vi "Periodic Tasks.vi"(8 "error in":errorcluster) -> ()   [LabVIEW 2013]
doc: "This VI runs in parallel to other tasks. It can contain as many user-defined periodic loops as you need. These can carry out PID or other sorts of timed response."
uses:
  <vilib>/Rock Robotics/SystemInterfaces/Utilities/FPGA_UtilitiesLED Source.ctl
  <vilib>/Rock Robotics/SystemInterfaces/Utilities/FPGA_UtilitiesLED State.ctl
  <vilib>/Rock Robotics/WPI/Joystick/WPI_JoystickGetSetRefNum.vi
  Robot Global Data.vi
  <vilib>/Rock Robotics/WPI/Relay/WPI_RelayValue.ctl
panel:
  out "JS Buttons 2":T1
  out "JS Buttons 1":T1
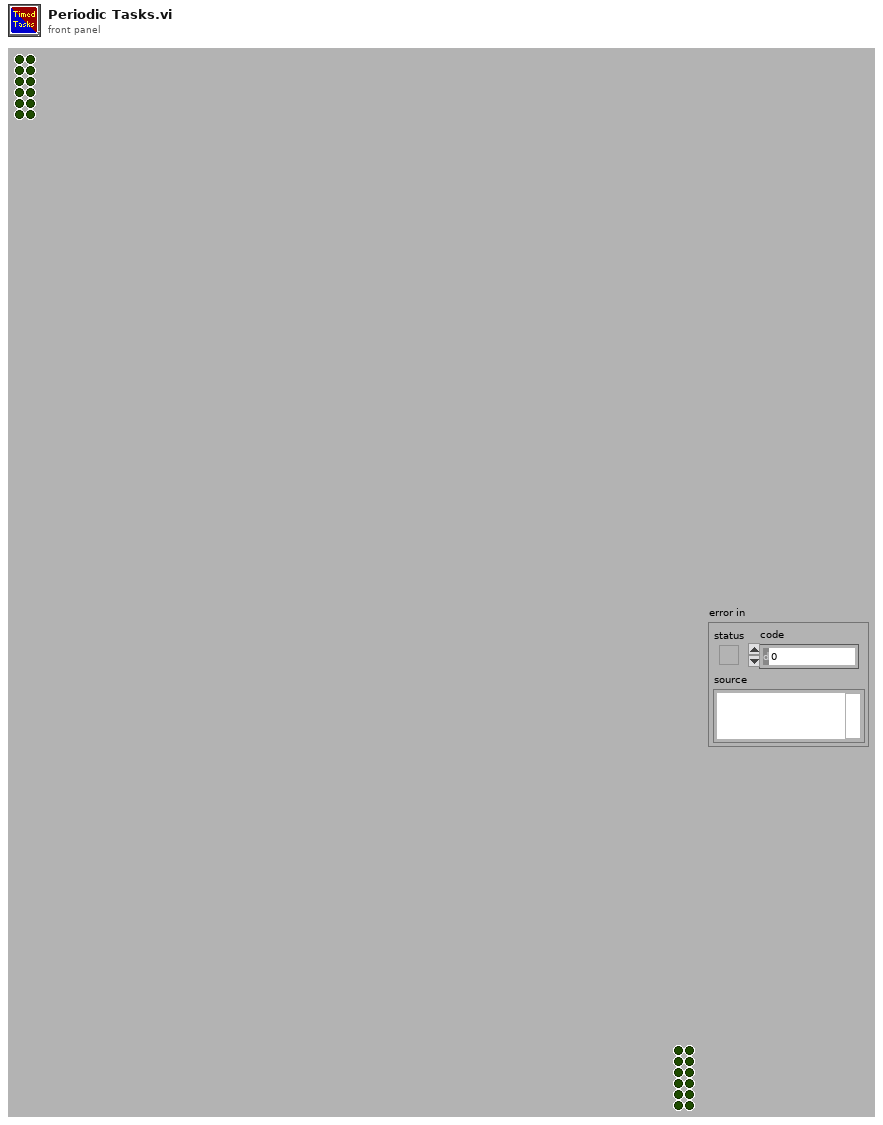
[diagram p1: front panel]
types:
  T1 = cluster{bool, bool, bool, bool, bool, bool, bool, bool, bool, bool, bool, bool}
  T2 = typedef "WPI_JoystickDevRef.ctl" = cluster{"Device":T3}
  T3 = typedef "WPI_JoystickDeviceEnum.ctl" = enum16{"USB 1", "USB 2", "USB 3", "USB 4", "Kinect 1", "Kinect 2"}
  T4 = typedef "WPI_ServoDeviceRef.ctl" = cluster{"DeviceStatus":errorcluster, "Digital Module":T5, "PWM Channel":T6, "DeadBand":T7}
  T5 = typedef "FPGA_TypedefDigitalModule.ctl" = enum16{"Digital Module 1", "Digital Module 2"}
  T6 = typedef "FPGA_DIOPWMChannel.ctl" = enum8{"PWM 1", "PWM 2", "PWM 3", "PWM 4", "PWM 5", "PWM 6", "PWM 7", "PWM 8", "PWM 9", "PWM 10", "Invalid"}
  T7 = typedef "WPI_PWMDeadband.ctl" = cluster{"Name":string, "maxPositivePwm":i32, "minPositivePwm":i32, "centerPwm":i32, "maxNegativePwm":i32, "minNegativePwm":i32, "angularRange":u16}
  T8 = typedef "WPI_MotorControlDeviceRef.ctl" = cluster{"DeviceStatus":errorcluster, "Type":enum16{"PWM", "CAN"}, "PWM":cluster{"Digital Module":T5, "PWM Channel":T6, "DeadBand":T7}, "CAN":cluster{"Device Number":u8, "Control Mode":T9, "Semaphore":T10, "Max Vout":dbl}, "Invert":bool, "TransformRef":T11, "InvTransformRef":T11}
  T9 = typedef "WPI_CANJaguar_ControlMode.ctl" = enum8{"Percent VBus", "Current", "Speed", "Position", "Voltage"}
  T10 = typedef "Semaphore RefNum" = refnum<k1>
  T11 = typedef "WPI_PWMTransform_ConPane.ctl" = refnum<vi>
  T12 = typedef "WPI_RelayDevRef.ctl" = cluster{"DevStatus":errorcluster, "Relay Channel":T13, "Digital Module":T5, "Relay Direction":T14}
  T13 = typedef "FPGA_DIORelayChannel.ctl" = enum8{"Relay 1", "Relay 2", "Relay 3", "Relay 4", "Relay 5", "Relay 6", "Relay 7", "Relay 8", "Invalid"}
  T14 = typedef "WPI_RelayDirection.ctl" = enum16{"Both directions", "Forward only", "Reverse only"}
  T15 = typedef "FPGA_UtilitiesLED State.ctl" = enum16{"Off", "On", "Toggle"}
  T16 = typedef "FPGA_UtilitiesLED Source.ctl" = enum16{"User LED", "FPGA LED"}
  T17 = typedef "WPI_RelayValue.ctl" = enum16{"Off", "On", "Forward", "Reverse"}
  T18 = typedef "WPI_JoystickButtonState.ctl" = cluster{"Button 1":bool, "Button 2":bool, "Button 3":bool, "Button 4":bool, "Button 5":bool, "Button 6":bool, "Button 7":bool, "Button 8":bool, "Button 9":bool, "Button 10":bool, "Button 11":bool, "Button 12":bool}
  T19 = cluster{"axis 1 (x)":dbl, "axis 2 (y)":dbl, "axis 3 (throttle)":dbl, "axis 4":dbl, "axis 5":dbl, "axis 6":dbl}
  T20 = typedef "WPI_DigitalInputDevRef.ctl" = cluster{"DevStatus":errorcluster, "DIO Channel":T21, "Digital Module":T5}
  T21 = typedef "FPGA_DIOChannel.ctl" = enum8{"DIO 1", "DIO 2", "DIO 3", "DIO 4", "DIO 5", "DIO 6", "DIO 7", "DIO 8", "DIO 9", "DIO 10", "DIO 11", "DIO 12", "DIO 13", "DIO 14", "Invalid"}
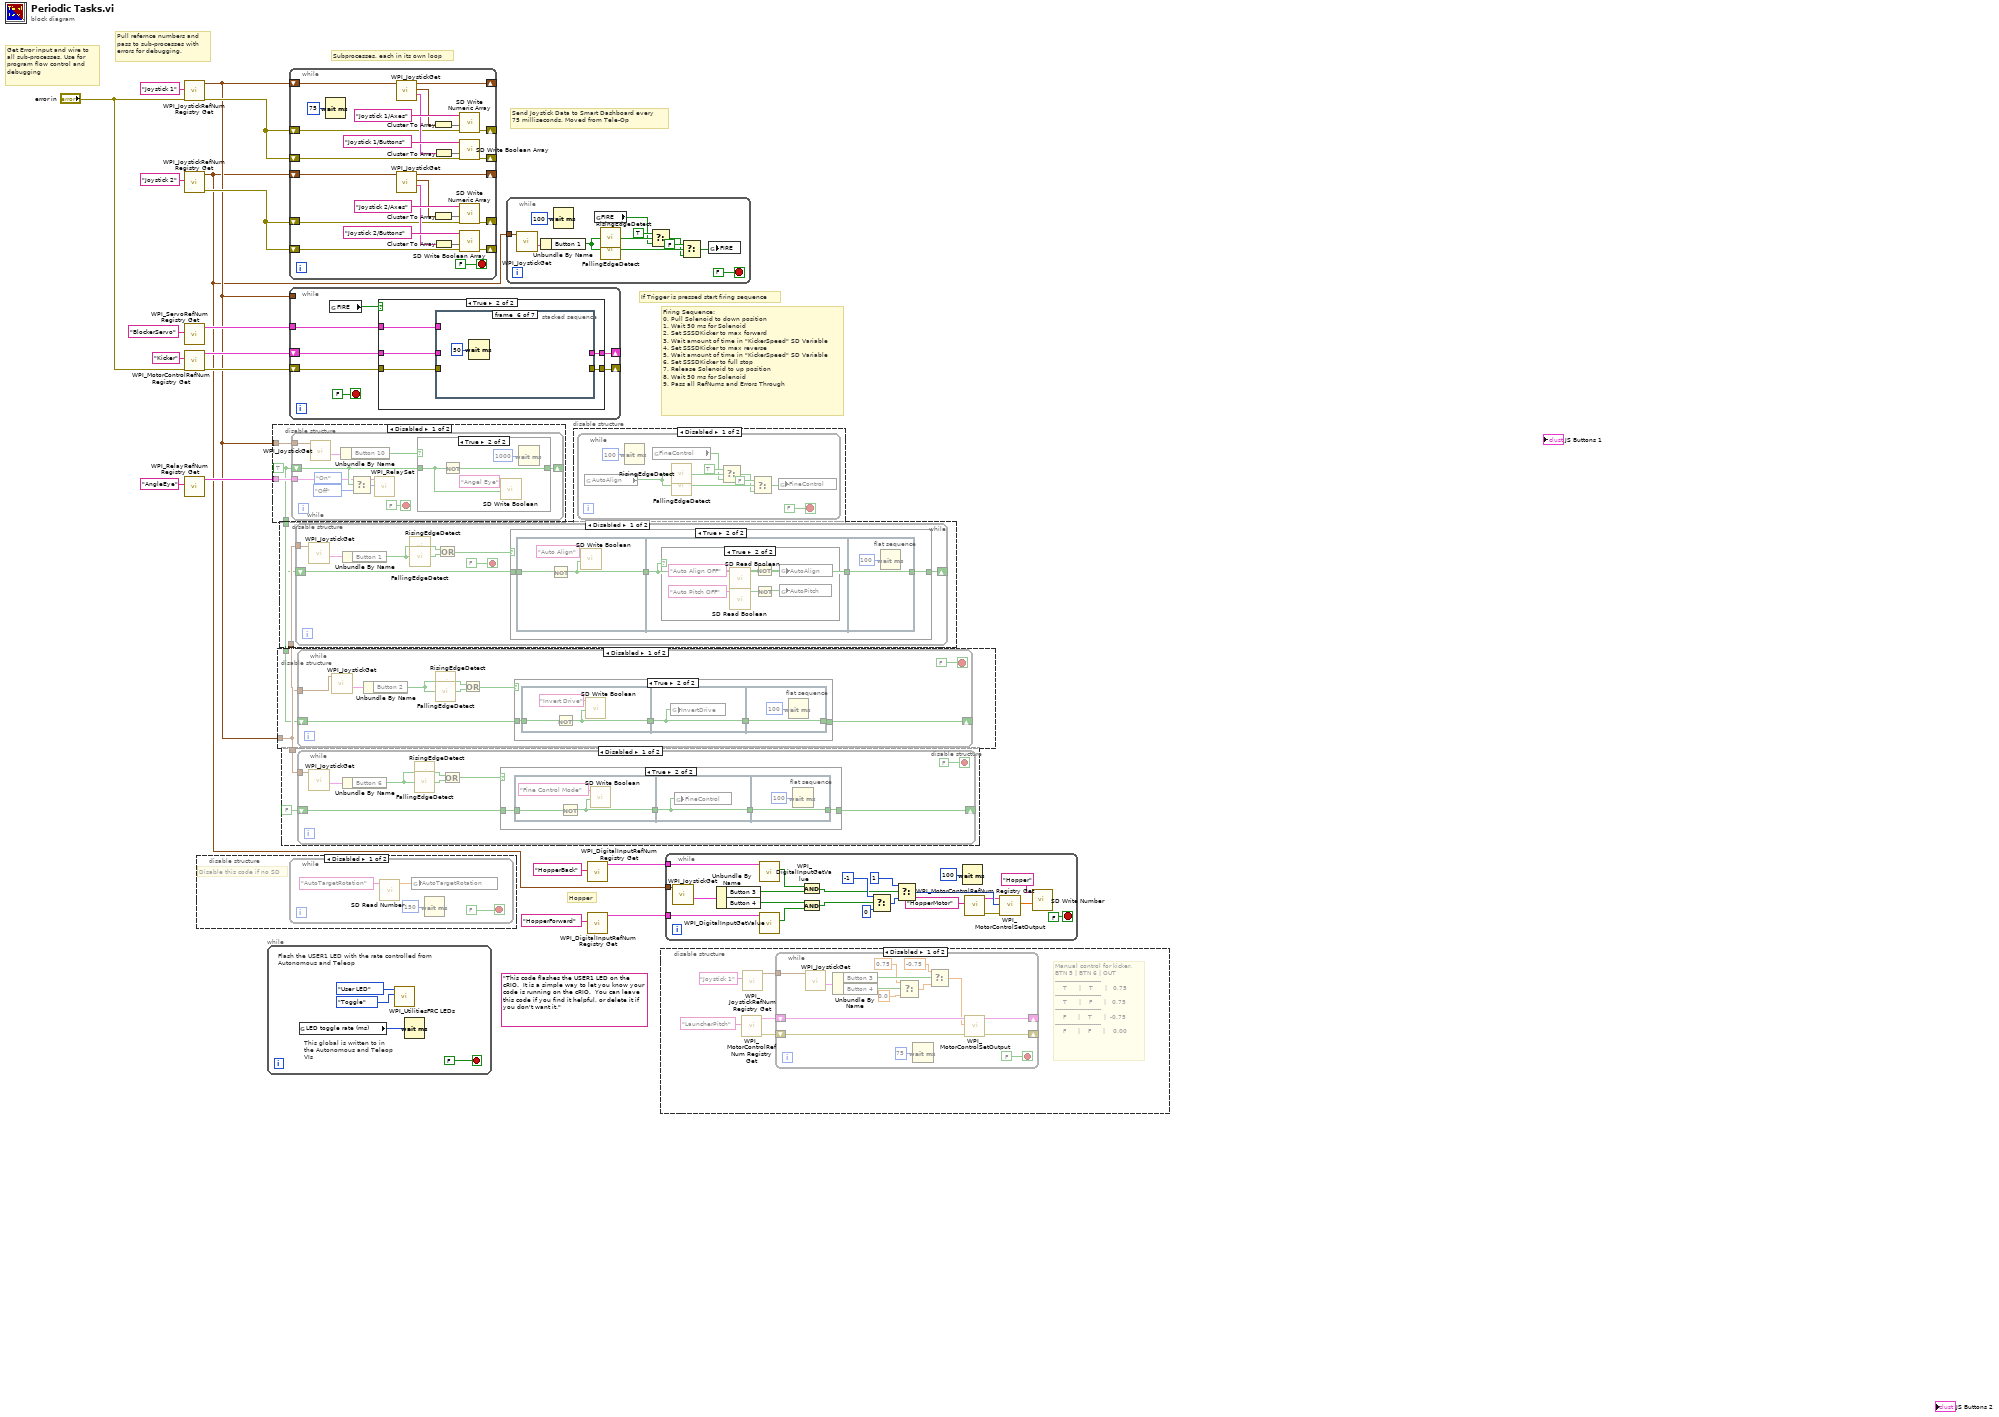
[diagram p0: block diagram]
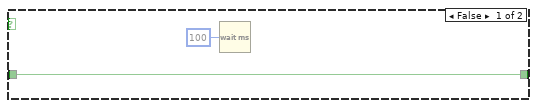
[diagram p3: hidden frame]
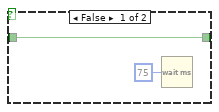
[diagram p5: hidden frame]
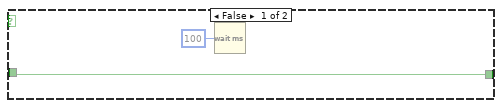
[diagram p7: hidden frame]
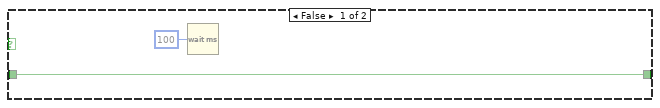
[diagram p11: hidden frame]
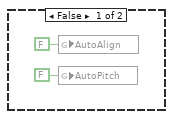
[diagram p12: hidden frame]
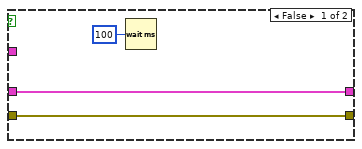
[diagram p14: hidden frame]
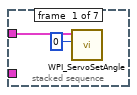
[diagram p15: hidden frame]
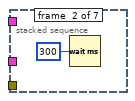
[diagram p16: hidden frame]
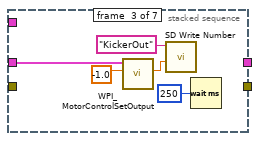
[diagram p17: hidden frame]
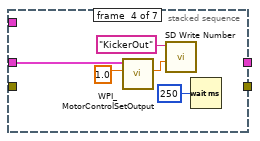
[diagram p18: hidden frame]
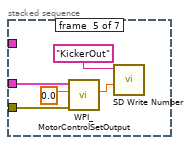
[diagram p19: hidden frame]
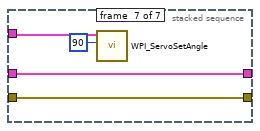
[diagram p20: hidden frame]
diagram:
  (unwired) "This code flashes the USER1 LED on the cRIO.  It is a simple way to let you know your code is running on the cRIO.  You can leave this code if you find it helpful, or delete it if you don't want it."
  # "Hopper"
  # "Firing Sequence:\n0. Pull Solenoid to down position\n1. Wait 50 ms for Solenoid\n2. Set SSSDKicker to max forward\n3. Wait amount of time in \"KickerSpeed\" SD Variable\n4. Set SSSDKicker to max reverse\n5. Wait amount of time in \"KickerSpeed\" SD Variable\n6. Set SSSDKicker to full stop\n7. Release Solenoid to up position\n8. Wait 50 ms for Solenoid\n9. Pass all RefNums and Errors Through"
  # "If Trigger is pressed start firing sequence"
  # "Subprocesses, each in its own loop"
  # "Pull refernce numbers and\npass to sub-processes with\nerrors for debugging."
  # "Get Error input and wire to\nall sub-processes. Use for\nprogram flow control and\ndebugging"
  # "Send Joystick Data to Smart Dashboard every\n75 milliseconds. Moved from Tele-Op"
  n1 = call <vilib>:"WPI_JoystickRefNum Registry Get.vi"("error in (no error)"="error in", "refnum name"="Joystick 1") -> ("error out"=w14:errorcluster, "JoystickDevRef"=w2:T2)  [unwired: 8 out]
  n2 = call <vilib>:"WPI_JoystickRefNum Registry Get.vi"("refnum name"="Joystick 2") -> ("error out"=w13:errorcluster, "JoystickDevRef"=w1:T2)  [unwired: 1 in, 8 out]
  n3 = call <vilib>:"WPI_ServoRefNum Registry Get.vi"("refnum name"="BlockerServo") -> ("ServoDeviceRef"=w9:T4)  [unwired: 9 in, 1 out]
  n4 = call <vilib>:"WPI_MotorControlRefNum Registry Get.vi"("error in (no error)"="error in", "refnum name"="Kicker") -> ("error out"=w17:errorcluster, "MotorControlDevRef"=w16:T8)  [unwired: 8 in]
  n5 = call <vilib>:"WPI_RelayRefNum Registry Get.vi"("refnum name"="AngleEye") -> ("RelayDevRef"=w11:T12)  [unwired: 9 in, 1 out]
  n6 = disable-structure shown="Disabled" {
    frame Disabled {
      # "Disable this code if no SD"
      n7 = while {
        stop <- FALSE stop-if-true
        n8 = call <vilib>:"SD Read Number.vi"("Name"="AutoTargetRotation") -> ("Numeric"=w21:dbl)  [unwired: 8 in, 2 out]
        n9 = global write "Robot Global Data.vi" "AutoTargetRotation"(w21) -> ()
        n10 = Wait (ms)(milliseconds to wait=u32 150) -> ()  [unwired: 1 out]
      }
    }
    frame Enabled {
    }
  }
  n11 = while {
    stop <- FALSE stop-if-true
    # "This global is written to in the Autonomous and Teleop VIs"
    # "Flash the USER1 LED with the rate controlled from Autonomous and Teleop"
    n12 = global read "Robot Global Data.vi" "LED toggle rate (ms)"() -> (w24:u32)
    n13 = call <vilib>:"WPI_UtilitiesFRC LEDs.vi"("State"=FPGA_UtilitiesLED_State."Toggle", "LED Type"=FPGA_UtilitiesLED_Source."User LED") -> ()  [unwired: 1 in, 9 out]
    n14 = Wait (ms)(milliseconds to wait=w24) -> ()  [unwired: 1 out]
  }
  n15 = disable-structure shown="Disabled" {
    disable-tunnel: w11 -> [w30 _]
    disable-tunnel: [w29 _] -> w3
    disable-tunnel: w2 -> [w28 _]
    frame Disabled {
      w29 = TRUE
      n16 = while {
        tunnel: w30 -> [w39]
        tunnel: w28 -> [w38]
        shift-right: [w32] -> _
        shift-left: w29 -> [w40]
        stop <- FALSE stop-if-true
        n17 = call <vilib>:"WPI_JoystickGet.vi"("JoystickDevRef"=w38) -> ("Buttons"=w33:T18)  [unwired: 4 in, 2 out]
        n18 = Unbundle By Name(w33) -> ("Button 10"=w37:bool)
        n19 = Select(t=WPI_RelayValue."On" ("RelayValue"), s=w40, f=WPI_RelayValue."Off" ("RelayValue")) -> (s? t:f=w36:T17)
        n20 = call <vilib>:"WPI_RelaySet.vi"("RelayValue"=w36, "RelayDevRef"=w39) -> ()  [unwired: 8 in, 2 out]
        n21 = case shown="True" w37 {
          tunnel: w40 -> [w41 w43]
          tunnel: [w41 w46] -> w32
          frame False {
            n22 = Wait (ms)(milliseconds to wait=u32 75) -> ()  [unwired: 1 out]
          }
          frame True {
            n23 = Not(x=w43) -> (.not. x?=w46:bool)
            n24 = call <vilib>:"SD Write Boolean.vi"("Boolean"=w43, "Name"="Angel Eye") -> ()  [unwired: 8 in, 2 out]
            n25 = Wait (ms)(milliseconds to wait=u32 1000) -> ()  [unwired: 1 out]
          }
        }
      }
    }
    frame Enabled {
    }
  }
  n26 = disable-structure shown="Disabled" {
    disable-tunnel: w3 -> [w48 _]
    disable-tunnel: w2 -> [w47 _]
    frame Disabled {
      n27 = while {
        tunnel: w47 -> [w52]
        shift-right: [w50] -> _
        shift-left: w48 -> [w49]
        stop <- FALSE stop-if-true
        n28 = call <vilib>:"WPI_JoystickGet.vi"("JoystickDevRef"=w52) -> ("Buttons"=w53:T18)  [unwired: 4 in, 2 out]
        n29 = Unbundle By Name(w53) -> ("Button 2"=w54:bool)
        n30 = call "RisingEdgeDetect.vi"("Input"=w54) -> ("Output"=w56:bool)
        n31 = call "FallingEdgeDetect.vi"("Input"=w54) -> ("Output"=w55:bool)
        n32 = Or(x=w56, y=w55) -> (x .or. y?=w57:bool)
        n33 = case shown="True" w57 {
          tunnel: [w58 w60] -> w50
          tunnel: w49 -> [w58 w61]
          frame False {
            n34 = Wait (ms)(milliseconds to wait=u32 100) -> ()  [unwired: 1 out]
          }
          frame True {
            n35 = flat-sequence {
              tunnel: w61 -> [w66]
              tunnel: [w64] -> w63
              tunnel: w63 -> [w67]
              tunnel: [w67] -> w62
              tunnel: [w69] -> w60
              tunnel: w62 -> [w69]
              frame #0 {
                n36 = Not(x=w66) -> (.not. x?=w64:bool)
                n37 = call <vilib>:"SD Write Boolean.vi"("Boolean"=w64, "Name"="Invert Drive") -> ()  [unwired: 8 in, 2 out]
              }
              frame #1 {
                n38 = global write "Robot Global Data.vi" "InvertDrive"(w67) -> ()
              }
              frame #2 {
                n39 = Wait (ms)(milliseconds to wait=u32 100) -> ()  [unwired: 1 out]
              }
            }
          }
        }
      }
    }
    frame Enabled {
    }
  }
  n40 = disable-structure shown="Disabled" {
    disable-tunnel: w2 -> [w71 _]
    disable-tunnel: w3 -> [w70 _]
    frame Disabled {
      n41 = while {
        tunnel: w71 -> [w74]
        shift-right: [w72] -> _
        shift-left: w70 -> [w80]
        stop <- FALSE stop-if-true
        n42 = call <vilib>:"WPI_JoystickGet.vi"("JoystickDevRef"=w74) -> ("Buttons"=w75:T18)  [unwired: 4 in, 2 out]
        n43 = Unbundle By Name(w75) -> ("Button 1"=w79:bool)
        n44 = call "RisingEdgeDetect.vi"("Input"=w79) -> ("Output"=w77:bool)
        n45 = call "FallingEdgeDetect.vi"("Input"=w79) -> ("Output"=w76:bool)
        n46 = Or(x=w77, y=w76) -> (x .or. y?=w78:bool)
        n47 = case shown="True" w78 {
          tunnel: w80 -> [w81 w86]
          tunnel: [w81 w85] -> w72
          frame False {
            n48 = Wait (ms)(milliseconds to wait=u32 100) -> ()  [unwired: 1 out]
          }
          frame True {
            n49 = flat-sequence {
              tunnel: w86 -> [w89]
              tunnel: [w87] -> w84
              tunnel: w84 -> [w90]
              tunnel: [w90] -> w83
              tunnel: [w100] -> w85
              tunnel: w83 -> [w100]
              frame #0 {
                n50 = Not(x=w89) -> (.not. x?=w87:bool)
                n51 = call <vilib>:"SD Write Boolean.vi"("Boolean"=w87, "Name"="Auto Align") -> ()  [unwired: 8 in, 2 out]
              }
              frame #1 {
                n52 = case shown="True" w90 {
                  frame False {
                    n53 = global write "Robot Global Data.vi" "AutoAlign"(FALSE ("AutoAlign")) -> ()
                    n54 = global write "Robot Global Data.vi" "AutoPitch"(FALSE ("AutoPitch")) -> ()
                  }
                  frame True {
                    n55 = call <vilib>:"SD Read Boolean.vi"("Name"="Auto Align OFF") -> ("Boolean"=w95:bool)  [unwired: 8 in, 2 out]
                    n56 = call <vilib>:"SD Read Boolean.vi"("Name"="Auto Pitch OFF") -> ("Boolean"=w93:bool)  [unwired: 8 in, 2 out]
                    n57 = Not(x=w95) -> (.not. x?=w96:bool)
                    n58 = Not(x=w93) -> (.not. x?=w94:bool)
                    n59 = global write "Robot Global Data.vi" "AutoAlign"(w96) -> ()
                    n60 = global write "Robot Global Data.vi" "AutoPitch"(w94) -> ()
                  }
                }
              }
              frame #2 {
                n61 = Wait (ms)(milliseconds to wait=u32 100) -> ()  [unwired: 1 out]
              }
            }
          }
        }
      }
    }
    frame Enabled {
    }
  }
  n62 = disable-structure shown="Disabled" {
    disable-tunnel: w2 -> [w101 _]
    frame Disabled {
      n63 = while {
        shift-right: [w103] -> _
        shift-left: FALSE -> [w108]
        tunnel: w101 -> [w105]
        stop <- FALSE stop-if-true
        n64 = call <vilib>:"WPI_JoystickGet.vi"("JoystickDevRef"=w105) -> ("Buttons"=w106:T18)  [unwired: 4 in, 2 out]
        n65 = Unbundle By Name(w106) -> ("Button 6"=w107:bool)
        n66 = call "RisingEdgeDetect.vi"("Input"=w107) -> ("Output"=w110:bool)
        n67 = call "FallingEdgeDetect.vi"("Input"=w107) -> ("Output"=w109:bool)
        n68 = Or(x=w110, y=w109) -> (x .or. y?=w111:bool)
        n69 = case shown="True" w111 {
          tunnel: w108 -> [w112 w114]
          tunnel: [w112 w115] -> w103
          frame False {
            n70 = Wait (ms)(milliseconds to wait=u32 100) -> ()  [unwired: 1 out]
          }
          frame True {
            n71 = flat-sequence {
              tunnel: [w119] -> w117
              tunnel: w114 -> [w118]
              tunnel: w117 -> [w121]
              tunnel: [w121] -> w116
              tunnel: [w123] -> w115
              tunnel: w116 -> [w123]
              frame #0 {
                n72 = Not(x=w118) -> (.not. x?=w119:bool)
                n73 = call <vilib>:"SD Write Boolean.vi"("Boolean"=w119, "Name"="Fine Control Mode") -> ()  [unwired: 8 in, 2 out]
              }
              frame #1 {
                n74 = global write "Robot Global Data.vi" "FineControl"(w121) -> ()
              }
              frame #2 {
                n75 = Wait (ms)(milliseconds to wait=u32 100) -> ()  [unwired: 1 out]
              }
            }
          }
        }
      }
    }
    frame Enabled {
    }
  }
  n76 = while {
    shift-right: [w140] -> _
    shift-left: w14 -> [w138]
    shift-right: [w139] -> _
    shift-left: w14 -> [w137]
    shift-right: [w136] -> _
    shift-left: w2 -> [w141]
    shift-right: [w124] -> _
    shift-left: w1 -> [w127]
    shift-right: [w126] -> _
    shift-left: w13 -> [w129]
    shift-right: [w125] -> _
    shift-left: w13 -> [w128]
    stop <- FALSE stop-if-true
    n77 = Wait (ms)(milliseconds to wait=u32 75) -> ()  [unwired: 1 out]
    n78 = call <vilib>:"WPI_JoystickGet.vi"("JoystickDevRef"=w141) -> ("Buttons"=w145:T18, "Axes"=w144:T19, "JoystickDevRef"=w136:T2)  [unwired: 1 in, 3 out]
    n79 = call <vilib>:"WPI_JoystickGet.vi"("JoystickDevRef"=w127) -> ("Buttons"=w131:T18, "Axes"=w130:T19, "JoystickDevRef"=w124:T2)  [unwired: 1 in, 3 out]
    n80 = Cluster To Array(cluster=w144) -> (array=w147:dbl[])
    n81 = Cluster To Array(cluster=w130) -> (array=w133:dbl[])
    n82 = Cluster To Array(cluster=w145) -> (array=w149:bool[])
    n83 = Cluster To Array(cluster=w131) -> (array=w135:bool[])
    n84 = call <vilib>:"SD Write Numeric Array.vi"("error in"=w138, "Numeric Array"=w147, "Name"="Joystick 1/Axes") -> ("error out"=w140:errorcluster)  [unwired: 7 in, 1 out]
    n85 = call <vilib>:"SD Write Boolean Array.vi"("error in"=w137, "Boolean Array"=w149, "Name"="Joystick 1/Buttons") -> ("error out"=w139:errorcluster)  [unwired: 7 in, 1 out]
    n86 = call <vilib>:"SD Write Numeric Array.vi"("error in"=w129, "Numeric Array"=w133, "Name"="Joystick 2/Axes") -> ("error out"=w126:errorcluster)  [unwired: 7 in, 1 out]
    n87 = call <vilib>:"SD Write Boolean Array.vi"("error in"=w128, "Boolean Array"=w135, "Name"="Joystick 2/Buttons") -> ("error out"=w125:errorcluster)  [unwired: 7 in, 1 out]
  }
  n88 = while {
    shift-right: [w153] -> _
    shift-left: w16 -> [w155]
    shift-right: [w152] -> _
    shift-left: w17 -> [w154]
    tunnel: w2 -> [_]
    tunnel: w9 -> [w151]
    stop <- FALSE stop-if-true
    n89 = global read "Robot Global Data.vi" "FIRE"() -> (w150:bool)
    n90 = case shown="True" w150 {
      tunnel: w155 -> [w158 w164]
      tunnel: w154 -> [w157 w163]
      tunnel: [w158 w162] -> w153
      tunnel: [w157 w161] -> w152
      tunnel: w151 -> [_ w160]
      frame False {
        n91 = Wait (ms)(milliseconds to wait=u32 100) -> ()  [unwired: 1 out]
      }
      frame True {
        n92 = stacked-sequence {
          tunnel: w164 -> [_ _ w172 w177 w181 _ w187]
          tunnel: w163 -> [_ _ _ _ w182 _ w186]
          tunnel: [_ _ _ _ _ _ w187] -> w162
          tunnel: [_ _ _ _ _ _ w186] -> w161
          tunnel: w160 -> [w166 _ _ _ _ _ w184]
          frame #0 {
            n93 = call <vilib>:"WPI_ServoSetAngle.vi"("Angle"=0, "ServoDeviceRef"=w166) -> ()  [unwired: 8 in, 2 out]
          }
          frame #1 {
            n94 = Wait (ms)(milliseconds to wait=u32 300) -> ()  [unwired: 1 out]
          }
          frame #2 {
            n95 = call <vilib>:"WPI_MotorControlSetOutput.vi"("Output"=-1.0, "MotorControlDevRef"=w172) -> ("Motor Output"=w168:dbl)  [unwired: 7 in, 2 out]
            n96 = call <vilib>:"SD Write Number.vi"("Numeric"=w168, "Name"="KickerOut") -> ()  [unwired: 8 in, 2 out]
            n97 = Wait (ms)(milliseconds to wait=u32 250) -> ()  [unwired: 1 out]
          }
          frame #3 {
            n98 = call <vilib>:"WPI_MotorControlSetOutput.vi"("Output"=1.0, "MotorControlDevRef"=w177) -> ("Motor Output"=w173:dbl)  [unwired: 7 in, 2 out]
            n99 = call <vilib>:"SD Write Number.vi"("Numeric"=w173, "Name"="KickerOut") -> ()  [unwired: 8 in, 2 out]
            n100 = Wait (ms)(milliseconds to wait=u32 250) -> ()  [unwired: 1 out]
          }
          frame #4 {
            n101 = call <vilib>:"WPI_MotorControlSetOutput.vi"("error in (no error)"=w182, "Output"=0.0, "MotorControlDevRef"=w181) -> ("Motor Output"=w178:dbl)  [unwired: 6 in, 2 out]
            n102 = call <vilib>:"SD Write Number.vi"("Numeric"=w178, "Name"="KickerOut") -> ()  [unwired: 8 in, 2 out]
          }
          frame #5 {
            n103 = Wait (ms)(milliseconds to wait=u32 50) -> ()  [unwired: 1 out]
          }
          frame #6 {
            n104 = call <vilib>:"WPI_ServoSetAngle.vi"("Angle"=90, "ServoDeviceRef"=w184) -> ()  [unwired: 8 in, 2 out]
          }
        }
      }
    }
  }
  n105 = while {
    tunnel: w1 -> [w189]
    stop <- FALSE stop-if-true
    n106 = call <vilib>:"WPI_JoystickGet.vi"("JoystickDevRef"=w189) -> ("Buttons"=w193:T18)  [unwired: 4 in, 2 out]
    n107 = Unbundle By Name(w193) -> ("Button 1"=w192:bool)
    n108 = Wait (ms)(milliseconds to wait=u32 100) -> ()  [unwired: 1 out]
    n109 = global read "Robot Global Data.vi" "FIRE"() -> (w191:bool)
    n110 = call "RisingEdgeDetect.vi"("Input"=w192) -> ("Output"=w199:bool)
    n111 = call "FallingEdgeDetect.vi"("Input"=w192) -> ("Output"=w196:bool)
    n112 = Select(t=TRUE, s=w199, f=w191) -> (s? t:f=w195:bool)
    n113 = Select(t=FALSE, s=w196, f=w195) -> (s? t:f=w190:bool)
    n114 = global write "Robot Global Data.vi" "FIRE"(w190) -> ()
  }
  n115 = disable-structure shown="Disabled" {
    frame Disabled {
      n116 = while {
        stop <- FALSE stop-if-true
        n117 = global read "Robot Global Data.vi" "AutoAlign"() -> (w200:bool)
        n118 = Wait (ms)(milliseconds to wait=u32 100) -> ()  [unwired: 1 out]
        n119 = global read "Robot Global Data.vi" "FineControl"() -> (w203:bool)
        n120 = call "RisingEdgeDetect.vi"("Input"=w200) -> ("Output"=w209:bool)
        n121 = call "FallingEdgeDetect.vi"("Input"=w200) -> ("Output"=w206:bool)
        n122 = Select(t=TRUE, s=w209, f=w203) -> (s? t:f=w205:bool)
        n123 = Select(t=FALSE, s=w206, f=w205) -> (s? t:f=w202:bool)
        n124 = global write "Robot Global Data.vi" "FineControl"(w202) -> ()
      }
    }
    frame Enabled {
    }
  }
  n125 = call <vilib>:"WPI_DigitalInputRefNum Registry Get.vi"("refnum name"="HopperBack") -> ("DigitalInputDevRef"=w5:T20)  [unwired: 9 in, 1 out]
  n126 = call <vilib>:"WPI_DigitalInputRefNum Registry Get.vi"("refnum name"="HopperForward") -> ("DigitalInputDevRef"=w4:T20)  [unwired: 9 in, 1 out]
  n127 = disable-structure shown="Disabled" {
    frame Disabled {
      # "Manual control for kicker.\nBTN 5 | BTN 6 | OUT\n-----------------------\n    T      |    T      |   0.75\n-----------------------\n    T      |    F      |   0.75\n-----------------------\n    F      |    T      |  -0.75\n-----------------------\n    F      |    F      |    0.00"
      n128 = call <vilib>:"WPI_MotorControlRefNum Registry Get.vi"("refnum name"="LauncherPitch") -> ("error out"=w213:errorcluster, "MotorControlDevRef"=w214:T8)  [unwired: 9 in]
      n129 = call <vilib>:"WPI_JoystickRefNum Registry Get.vi"("refnum name"="Joystick 1") -> ("JoystickDevRef"=w210:T2)  [unwired: 1 in, 9 out]
      n130 = while {
        tunnel: w210 -> [w227]
        shift-right: [w216] -> _
        shift-left: w214 -> [w229]
        shift-right: [w215] -> _
        shift-left: w213 -> [w228]
        stop <- FALSE stop-if-true
        n131 = call <vilib>:"WPI_JoystickGet.vi"("JoystickDevRef"=w227) -> ("Buttons"=w226:T18)  [unwired: 4 in, 2 out]
        n132 = Unbundle By Name(w226) -> ("Button 3"=w225:bool, "Button 4"=w224:bool)
        n133 = Select(t=0.75, s=w224, f=0.0) -> (s? t:f=w223:dbl)
        n134 = Wait (ms)(milliseconds to wait=u32 75) -> ()  [unwired: 1 out]
        n135 = Select(t=-0.75, s=w225, f=w223) -> (s? t:f=w222:dbl)
        n136 = call <vilib>:"WPI_MotorControlSetOutput.vi"("error in (no error)"=w228, "Output"=w222, "MotorControlDevRef"=w229) -> ("error out"=w215:errorcluster, "MotorControlDevRef"=w216:T8)  [unwired: 6 in, 1 out]
      }
    }
    frame Enabled {
    }
  }
  n137 = while {
    tunnel: w1 -> [w240]
    tunnel: w5 -> [w235]
    tunnel: w4 -> [w234]
    stop <- FALSE stop-if-true
    n138 = call <vilib>:"WPI_JoystickGet.vi"("JoystickDevRef"=w240) -> ("Buttons"=w241:T18)  [unwired: 4 in, 2 out]
    n139 = Unbundle By Name(w241) -> ("Button 3"=w237:bool, "Button 4"=w236:bool)
    n140 = call <vilib>:"WPI_DigitalInputGetValue.vi"("DigitalInputDevRef"=w235) -> ("Value"=w230:bool)  [unwired: 8 in, 2 out]
    n141 = call <vilib>:"WPI_DigitalInputGetValue.vi"("DigitalInputDevRef"=w234) -> ("Value"=w231:bool)  [unwired: 8 in, 2 out]
    n142 = And(x=w230, y=w237) -> (x .and. y?=w233:bool)
    n143 = And(x=w236, y=w231) -> (x .and. y?=w232:bool)
    n144 = Select(t=-1, s=w232, f=0) -> (s? t:f=w249:i32)
    n145 = Select(t=1, s=w233, f=w249) -> (s? t:f=w251:i32)
    n146 = Wait (ms)(milliseconds to wait=u32 100) -> ()  [unwired: 1 out]
    n147 = call <vilib>:"WPI_MotorControlRefNum Registry Get.vi"("refnum name"="HopperMotor") -> ("error out"=w243:errorcluster, "MotorControlDevRef"=w242:T8)  [unwired: 9 in]
    n148 = call <vilib>:"WPI_MotorControlSetOutput.vi"("error in (no error)"=w243, "Output"=w251, "MotorControlDevRef"=w242) -> ("Motor Output"=w245:dbl)  [unwired: 6 in, 2 out]
    n149 = call <vilib>:"SD Write Number.vi"("Numeric"=w245, "Name"="Hopper") -> ()  [unwired: 8 in, 2 out]
  }
